vi "Jump Button Init.vi"(3 "Container State":T3, 4 "Previous State":variant, 5 "Previous Version":T2 {"Major" max=0; "Minor" max=0; "Fix" max=0; "Build" max=0}) -> (2 "Current State":T1)   [LabVIEW 2009, in "Jump Button (System).xctl"]
uses:
  <vilib>/Navigation Controls/Jump Button System/Jump Button (System).xctl
  <vilib>/Navigation Controls/Jump Button System/Jump Button State.ctl
  <vilib>/_xctls/Container State.ctl
  <vilib>/_xctls/Version.ctl
  <vilib>/Navigation Controls/NI_Navigation.lvlib
  <vilib>/_xctls/XControlSupport.lvlib
panel:
  in  "Failed to create":string="Error creating navigation button."
  in  "Default Indicator State":T1
  in  "Default Control State":T1
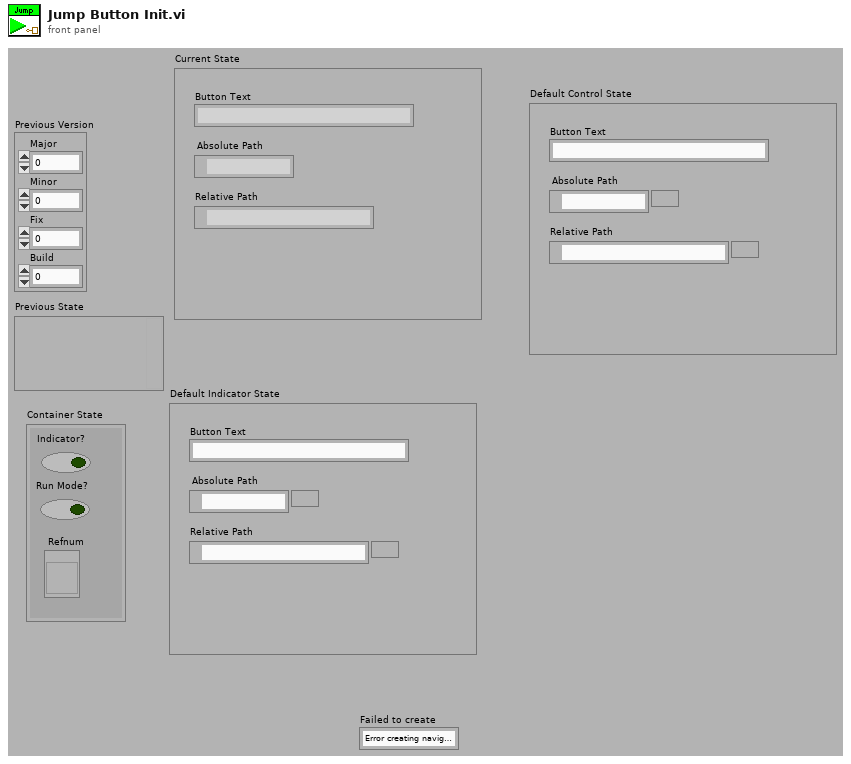
[diagram p1: front panel]
types:
  T1 = typedef "Jump Button (System).xctl/Jump Button State.ctl" = cluster{"Button Text":string, "Absolute Path":path, "Relative Path":path}
  T2 = typedef "XControlSupport.lvlib/Version.ctl" = cluster{"Major":u16, "Minor":u16, "Fix":u16, "Build":u16}
  T3 = typedef "XControlSupport.lvlib/Container State.ctl" = cluster{"Indicator?":bool, "Run Mode?":bool, " Refnum":refnum<vi>}
  T4 = enum32{"Next Modern", "Next System", "Previous Modern", "Previous System", "Jump Modern", "Jump System", "N/A"}
  T5 = cluster{"Button Text":string, "Absolute Path":path, "Relative Path":path}
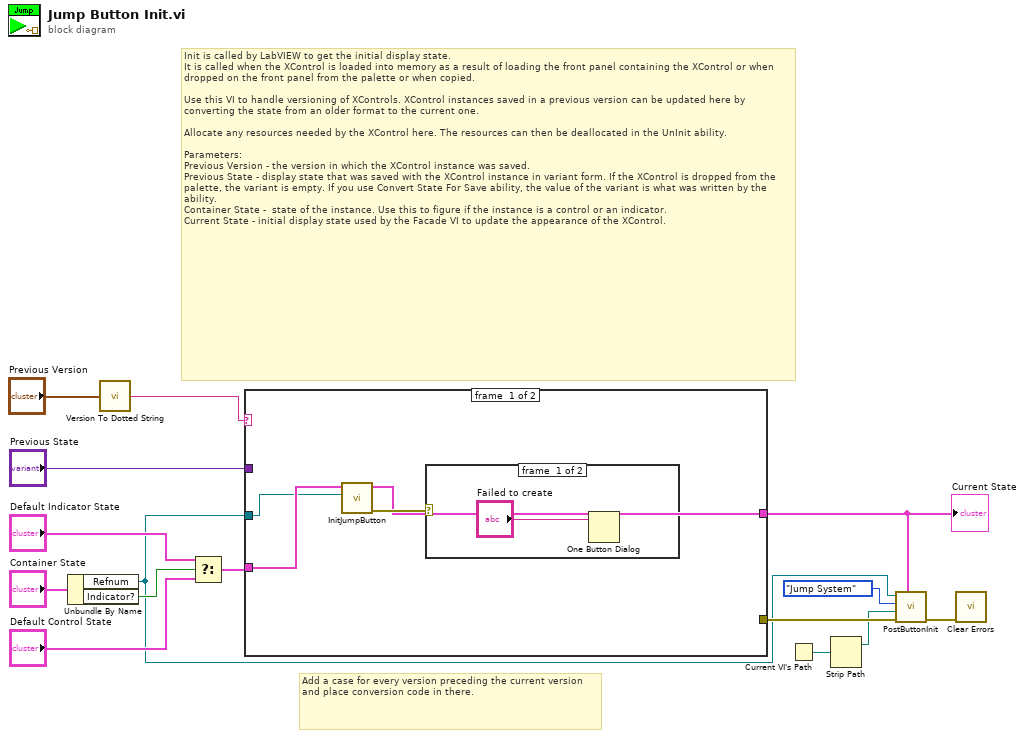
[diagram p0: block diagram]
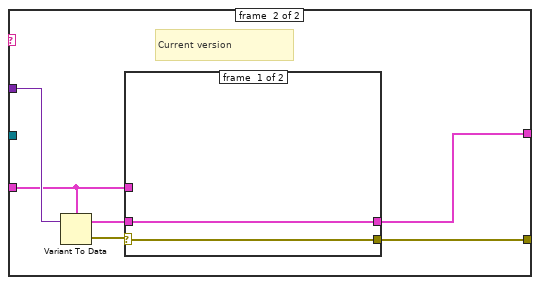
[diagram p3: hidden frame]
diagram:
  # "Add a case for every version preceding the current version and place conversion code in there."
  # "Init is called by LabVIEW to get the initial display state.\nIt is called when the XControl is loaded into memory as a result of loading the front panel containing the XControl or when dropped on the front panel from the palette or when copied.\n\nUse this VI to handle versioning of XControls. XControl instances saved in a previous version can be updated here by converting the state from an older format to the current one.\n\nAllocate any resources needed by the XControl here. The resources can then be deallocated in the UnInit ability.\n\nParameters:\nPrevious Version - the version in which the XControl instance was saved.\nPrevious State - display state that was saved with the XControl instance in variant form. If the XControl is dropped from the palette, the variant is empty. If you use Convert State For Save ability, the value of the variant is what was written by the ability. \nContainer State -  state of the instance. Use this to figure if the instance is a control or an indicator.\nCurrent State - initial display state used by the Facade VI to update the appearance of the XControl."
  n1 = Unbundle By Name("Container State") -> ("Refnum"=w1:refnum<vi>, "Indicator?"=w11:bool)
  n2 = call <vilib>:"Version To Dotted String.vi"("Version"="Previous Version") -> ("String Version"=w9:string)
  n3 = Select(t="Default Indicator State", s=w11, f="Default Control State") -> (s? t:f=w8:T1)
  n4 = case shown="\"0.0.0.0\"" w9 {
    tunnel: "Previous State" -> [_ w26]
    tunnel: [w18 w22] -> w3
    tunnel: w8 -> [w17 w23]
    tunnel: [_ w21] -> w7
    tunnel: w1 -> [w16 _]
    frame #0 {
      n5 = call <vilib>:"InitJumpButton.vi"("ctl reference"=w16, "default state"=w17) -> ("error out"=w19:errorcluster, "state out"=w18:T5)  [unwired: 8 in]
      n6 = case shown="Error" w19 {
        frame #0 {
          n7 = One Button Dialog(message="Failed to create") -> ()  [unwired: 1 in, 1 out]
        }
        frame #1 {
        }
      }
    }
    frame #1 {
      # "Current version"
      n8 = Variant To Data(Variant=w26, type=w23) -> (error out=w25:errorcluster, data=w24:T1)  [unwired: 1 in]
      n9 = case shown="No Error" w25 {
        selector: w25 -> [w28 w29]
        tunnel: w24 -> [w27 _]
        tunnel: [w27 w30] -> w22
        tunnel: w23 -> [_ w30]
        tunnel: [w28 w29] -> w21
        frame #0 {
        }
        frame #1 {
          # "Error converting previously \nsaved state. Use default instead."
        }
      }
    }
  }
  "Current State" <- w3
  n10 = Current VI's Path() -> (path=w5:path)
  n11 = Strip Path(path=w5) -> (stripped path=w4:path)  [unwired: 1 out]
  n12 = call <vilib>:"PostButtonInit.vi"("State"=w3, "error in (no error)"=w7, "Current Path"=w4, "Button Type"=T4."Jump System", "Control Refnum"=w1) -> ("error out"=w2:errorcluster)  [unwired: 5 in, 1 out]
  n13 = call <vilib>:"Clear Errors.vi"("error in (no error)"=w2) -> ()  [unwired: 6 in, 1 out]
